vi "Definite_time_function.vi"(6 "RMS minimum\nvalues":T7, 7 "input cluster":T3, 9 "RMS values":T6, 10 "Active Power":dbl[](array[numeric]), 11 "Protection settings":T5) -> (0 "I RMS":dbl, 1 "VR RMS":dbl, 2 "VL RMS":dbl, 3 "trip signal":bool, 4 "Blocking signal":bool[](array[boolean]), 5 "output cluster":T3)   [LabVIEW 2016]
uses:
  <vilib>/addons/Electrical Power/Protection/Definite Time Delay/subVIs/fpga_Time Delay Cfg.ctl
  <vilib>/addons/Electrical Power/Protection/Definite Time Delay/subVIs/fpga_Timer Feedback Var.ctl
  <vilib>/addons/Electrical Power/Protection/Definite Time Delay/subVIs/fpga_State.ctl
  <vilib>/addons/Electrical Power/Protection/NI_EP_Protection_FPGA.lvlib
panel:
  out "Direction":enum16{"forward", "backward", "N/D"}(ring)
  out "I error":i32
  out "VL error":i32
  out "VR error":i32
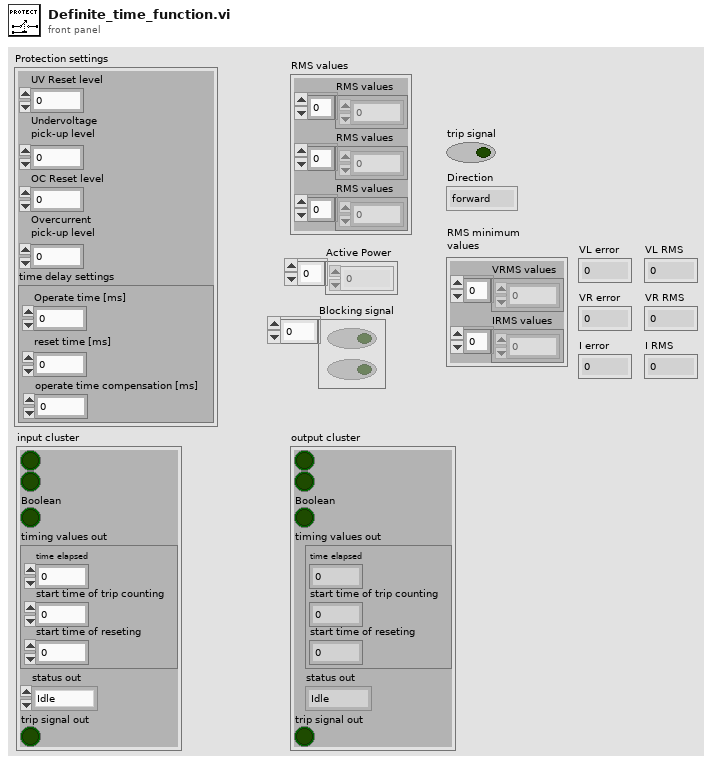
[diagram p1: front panel]
types:
  T1 = typedef "NI_EP_Protection_FPGA.lvlib/fpga_Timer Feedback Var.ctl" = cluster{"time elapsed":u32, "start time of trip counting":u32, "start time of reseting":u32}
  T2 = typedef "NI_EP_Protection_FPGA.lvlib/fpga_State.ctl" = enum16{"Idle", "Trip Counting", "Tripped", "Reset Counting"}
  T3 = cluster{bool, bool, "Boolean":bool, "timing values out":T1, "status out":T2, "trip signal out":bool}
  T4 = typedef "NI_EP_Protection_FPGA.lvlib/fpga_Time Delay Cfg.ctl" = cluster{"Operate time [ms]":u32, "reset time [ms]":u32, "operate time compensation [ms]":u32}
  T5 = cluster{"UV Reset level":dbl, "Undervoltage \npick-up level":dbl, "OC Reset level":dbl, "Overcurrent\npick-up level":dbl, "time delay settings":T4}
  T6 = cluster{"RMS values":dbl[], "RMS values":dbl[], "RMS values":dbl[]}
  T7 = cluster{"VRMS values":dbl[], "IRMS values":dbl[]}
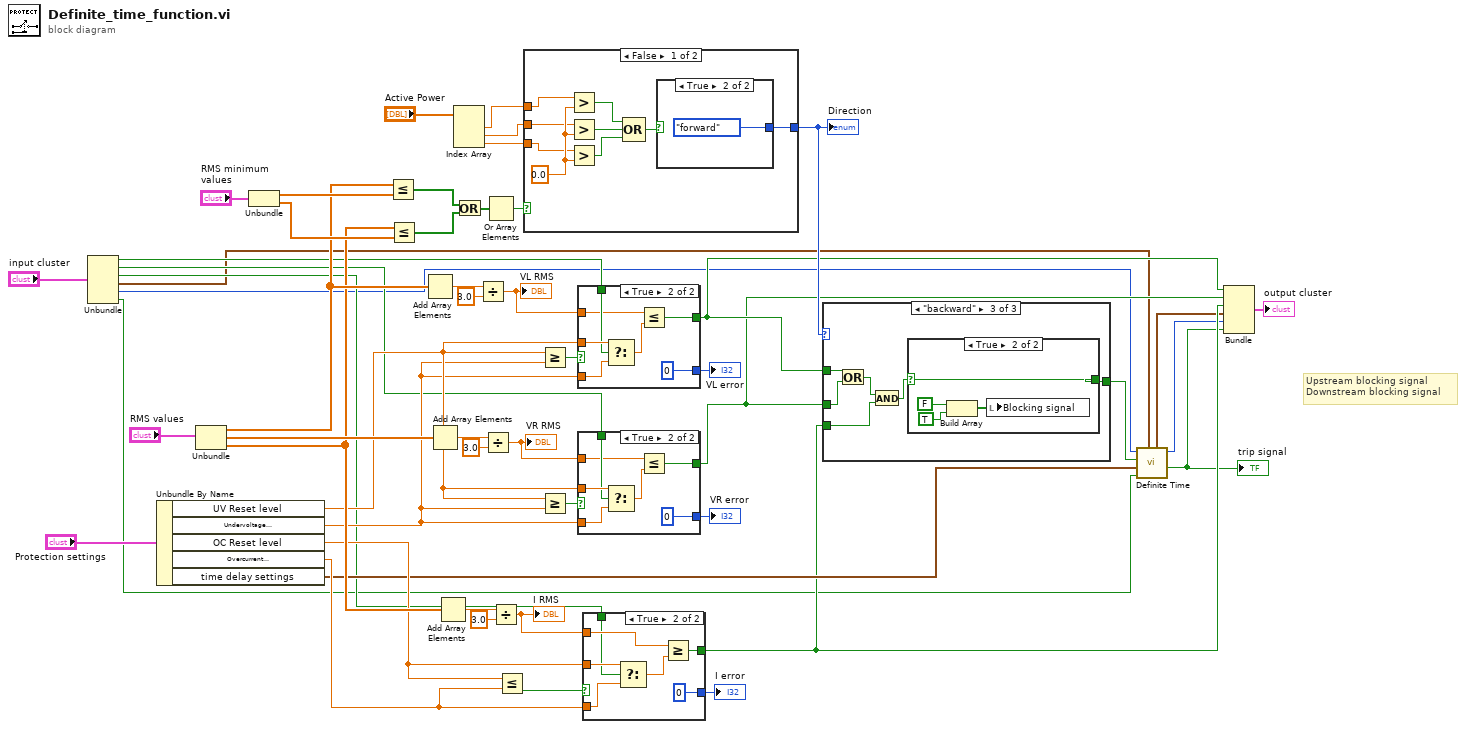
[diagram p0: block diagram]
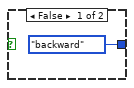
[diagram p2: hidden frame]
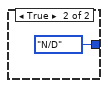
[diagram p3: hidden frame]
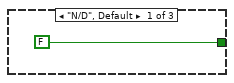
[diagram p4: hidden frame]
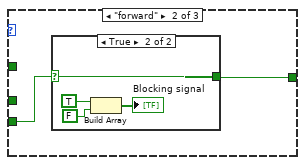
[diagram p5: hidden frame]
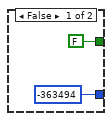
[diagram p8: hidden frame]
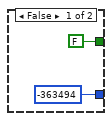
[diagram p9: hidden frame]
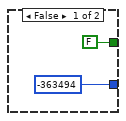
[diagram p10: hidden frame]
diagram:
  # "Upstream blocking signal\nDownstream blocking signal"
  n1 = Unbundle("input cluster") -> (w10:bool, w9:bool, "Boolean"=w8:bool, "timing values out"=w7:T1, "status out"=w6:T2, "trip signal out"=w5:bool)
  n2 = Unbundle By Name("Protection settings") -> ("UV Reset level"=w23:dbl, "Undervoltage \npick-up level"=w22:dbl, "OC Reset level"=w21:dbl, "Overcurrent\npick-up level"=w20:dbl, "time delay settings"=w19:T4)
  n3 = Unbundle("RMS values") -> ("RMS values"=w27:dbl[], "RMS values"=w26:dbl[], "RMS values"=w25:dbl[])
  n4 = Unbundle("RMS minimum\nvalues") -> ("VRMS values"=w44:dbl[], "IRMS values"=w38:dbl[])
  n5 = Less Or Equal?(x=w27, y=w44) -> (x <= y?=w43:bool[])
  n6 = Less Or Equal?(x=w25, y=w38) -> (x <= y?=w42:bool[])
  n7 = Add Array Elements(numeric array=w27) -> (sum=w37:dbl)
  n8 = Add Array Elements(numeric array=w26) -> (sum=w33:dbl)
  n9 = Add Array Elements(numeric array=w25) -> (sum=w30:dbl)
  n10 = Index Array(array="Active Power") -> (element #1=w3:dbl, element #2=w2:dbl, element #3=w1:dbl)  [unwired: 3 in]
  n11 = Or(x=w43, y=w42) -> (x .or. y?=w41:bool[])
  n12 = Divide(x=w37, y=3.0) -> (x/y=w35:dbl)
  "VL RMS" <- w35
  n13 = Divide(x=w33, y=3.0) -> (x/y=w32:dbl)
  "VR RMS" <- w32
  n14 = Or Array Elements(Boolean array=w41) -> (logical OR=w40:bool)
  n15 = Divide(x=w30, y=3.0) -> (x/y=w29:dbl)
  "I RMS" <- w29
  n16 = Less Or Equal?(x=w21, y=w20) -> (x <= y?=w52:bool)
  n17 = case shown="False" w40 {
    tunnel: w3 -> [w55 _]
    tunnel: w2 -> [w54 _]
    tunnel: w1 -> [w53 _]
    tunnel: [w56 enum16{"forward", "backward", "N/D"}."N/D"] -> w39
    frame False {
      w61 = 0.0 ("y")
      n18 = Greater?(x=w55, y=w61) -> (0:w60:bool)
      n19 = Greater?(x=w54, y=w61) -> (0:w59:bool)
      n20 = Greater?(x=w53, y=w61) -> (0:w58:bool)
      n21 = Compound Arithmetic op=OR(w60, w59, w58) -> (w57:bool)
      n22 = case shown="True" w57 {
        tunnel: [enum16{"forward", "backward", "N/D"}."backward" enum16{"forward", "backward", "N/D"}."forward"] -> w56
        frame False {
        }
        frame True {
        }
      }
    }
    frame True {
    }
  }
  "Direction" <- w39
  n23 = Greater Or Equal?(x=w23, y=w22) -> (x >= y?=w50:bool)
  n24 = Greater Or Equal?(x=w23, y=w22) -> (x >= y?=w47:bool)
  n25 = case shown="True" w50 {
    tunnel: [FALSE w72] -> w18
    tunnel: [-363494 ("error") 0 ("error")] -> w49
    tunnel: w23 -> [_ w70]
    tunnel: w22 -> [_ w69]
    tunnel: w10 -> [_ w68]
    tunnel: w35 -> [_ w67]
    frame False {
    }
    frame True {
      n26 = Select(t=w70, s=w68, f=w69) -> (s? t:f=w73:dbl)
      n27 = Less Or Equal?(x=w67, y=w73) -> (x <= y?=w72:bool)
    }
  }
  "VL error" <- w49
  n28 = case shown="True" w47 {
    tunnel: [FALSE w81] -> w17
    tunnel: [-363494 ("error") 0 ("error")] -> w48
    tunnel: w23 -> [_ w79]
    tunnel: w22 -> [_ w78]
    tunnel: w9 -> [_ w77]
    tunnel: w32 -> [_ w76]
    frame False {
    }
    frame True {
      n29 = Select(t=w79, s=w77, f=w78) -> (s? t:f=w82:dbl)
      n30 = Less Or Equal?(x=w76, y=w82) -> (x <= y?=w81:bool)
    }
  }
  "VR error" <- w48
  n31 = case shown="True" w52 {
    tunnel: w29 -> [_ w91]
    tunnel: [-363494 ("error") 0 ("error")] -> w51
    tunnel: w21 -> [_ w88]
    tunnel: w20 -> [_ w87]
    tunnel: [FALSE ("Boolean") w86] -> w16
    tunnel: w8 -> [_ w85]
    frame False {
    }
    frame True {
      n32 = Select(t=w88, s=w85, f=w87) -> (s? t:f=w90:dbl)
      n33 = Greater Or Equal?(x=w91, y=w90) -> (x >= y?=w86:bool)
    }
  }
  "I error" <- w51
  n34 = case shown="\"backward\"" w39 {
    tunnel: w18 -> [_ _ w105]
    tunnel: w17 -> [_ _ w104]
    tunnel: w16 -> [_ w94 w102]
    tunnel: [FALSE ("Boolean") w93 w101] -> w46
    frame "N/D", Default {
    }
    frame "forward" {
      n35 = case shown="True" w94 {
        selector: w94 -> [w95 w99]
        tunnel: [w95 w99] -> w93
        frame False {
        }
        frame True {
          n36 = Build Array(TRUE, FALSE) -> (→"Blocking signal":bool[])
        }
      }
    }
    frame "backward" {
      n37 = Or(x=w105, y=w104) -> (x .or. y?=w103:bool)
      n38 = And(x=w103, y=w102) -> (x .and. y?=w100:bool)
      n39 = case shown="True" w100 {
        selector: w100 -> [w106 w110]
        tunnel: [w106 w110] -> w101
        frame False {
        }
        frame True {
          n40 = Build Array(FALSE, TRUE) -> (w107:bool[])
          n41 = local write "Blocking signal"(w107) -> ()
        }
      }
    }
  }
  n42 = call "Definite Time.vi"("timing values in"=w7, "trip signal in"=w5, "time delay settings"=w19, "pick-up signal? (F)"=w46, "status in"=w6) -> ("trip signal out"=w13:bool, "status out"=w14:T2, "timing values out"=w15:T1)  [unwired: 4 in]
  "trip signal" <- w13
  n43 = Bundle(w18, w17, "Boolean"=w16, "timing values out"=w15, "status out"=w14, "trip signal out"=w13) -> (→"output cluster":T3)  [unwired: 1 in]
